vi "Stop Core.vi"(10 "final error code":i32 caption="最终错误代码", 11 "THM-V6数字型温湿度 in":refnum<class "THM-V6数字型温湿度.lvclass"> caption="操作者输入") -> (3 "THM-V6数字型温湿度 out":refnum<class "THM-V6数字型温湿度.lvclass"> caption="操作者输出")   [LabVIEW 2016, in "THM-V6数字型温湿度.lvlib" / "THM-V6数字型温湿度.lvclass"]
doc: "(<B>Filename</B>: Actor Framework.lvlib:Actor.lvclass:Stop Core.vi)\n\nDefines what the actor does before it stops. Use the <B>final error code</B> input to determine whether the actor shut down in response to an error.\n\nBy default, this method does nothing.子孙类重写该方法，定义出错时的操作，例如，关闭操作者核心方法初始的进程。"
uses:
  <vilib>/ActorFramework/Actor/Actor.lvclass
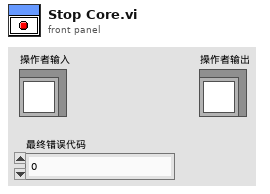
[diagram p1: front panel]
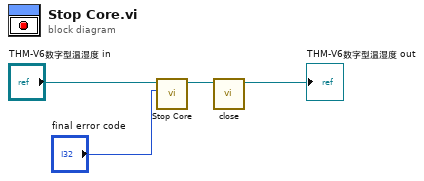
[diagram p0: block diagram]
diagram:
  n1 = call-parent "Stop Core.vi"("final error code"="final error code", "Actor in"="THM-V6数字型温湿度 in") -> ("Actor out"=w2:refnum<class "THM-V6数字型温湿度.lvclass">)  [unwired: 9 in]
  n2 = call "close.vi"("THM-V6数字型温湿度 输入"=w2) -> ("THM-V6数字型温湿度 输出"=→"THM-V6数字型温湿度 out":refnum<class "THM-V6数字型温湿度.lvclass">)  [unwired: 9 in, 1 out]
